vi "Check Message Data Clusters.vi"(8 "error in (no error)":errorcluster, 10 "Fields Data":T1[](array[typedef]), 11 "Message Data Cluster in":refnum<vi>) -> (0 "error out":errorcluster, 2 "Unmodified?":bool, 3 "Message Data Cluster out":refnum<vi>)   [LabVIEW 2019, in "gRPC Template Creation Utility.lvlib"]
uses:
  gRPC Template Creation Utility.lvlib
  TypeDefs/Message Element Metadata (Scripting).ctl
  TypeDefs/Message Element Type.ctl
  <vilib>/numeric/LVNumericRepresentation.ctl
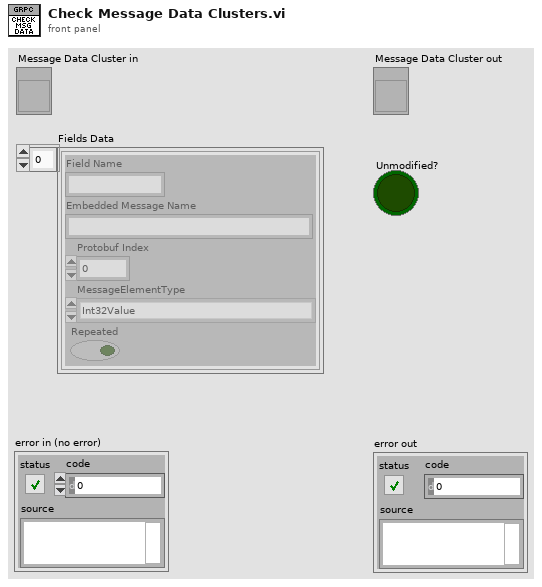
[diagram p1: front panel]
types:
  T1 = typedef "gRPC Template Creation Utility.lvlib/Message Element Metadata (Scripting).ctl" = cluster{"Field Name":string, "Embedded Message Name":string, "Protobuf Index":i32, "MessageElementType":T2, "Repeated":bool}
  T2 = typedef "gRPC Template Creation Utility.lvlib/Message Element Type.ctl" = enum32{"Int32Value", "FloatValue", "DoubleValue", "BoolValue", "StringValue", "MessageValue", "Int64Value", "UInt32Value", "UInt64Value", "EnumValue", "Bytes", "Fixed64", "Fixed32", "SFixed64", "SFixed32", "SInt64", "SInt32"}
  T3 = typedef "LVNumericRepresentation.ctl" = enum32{"Extended Precision", "Double Precision", "Single Precision", "Long", "Word", "Byte", "Unsigned Long", "Unsigned Word", "Unsigned Byte", "Complex Extended", "Complex Double", "Complex Single", "Quad", "Unsigned Quad", "Fixed-Point"}
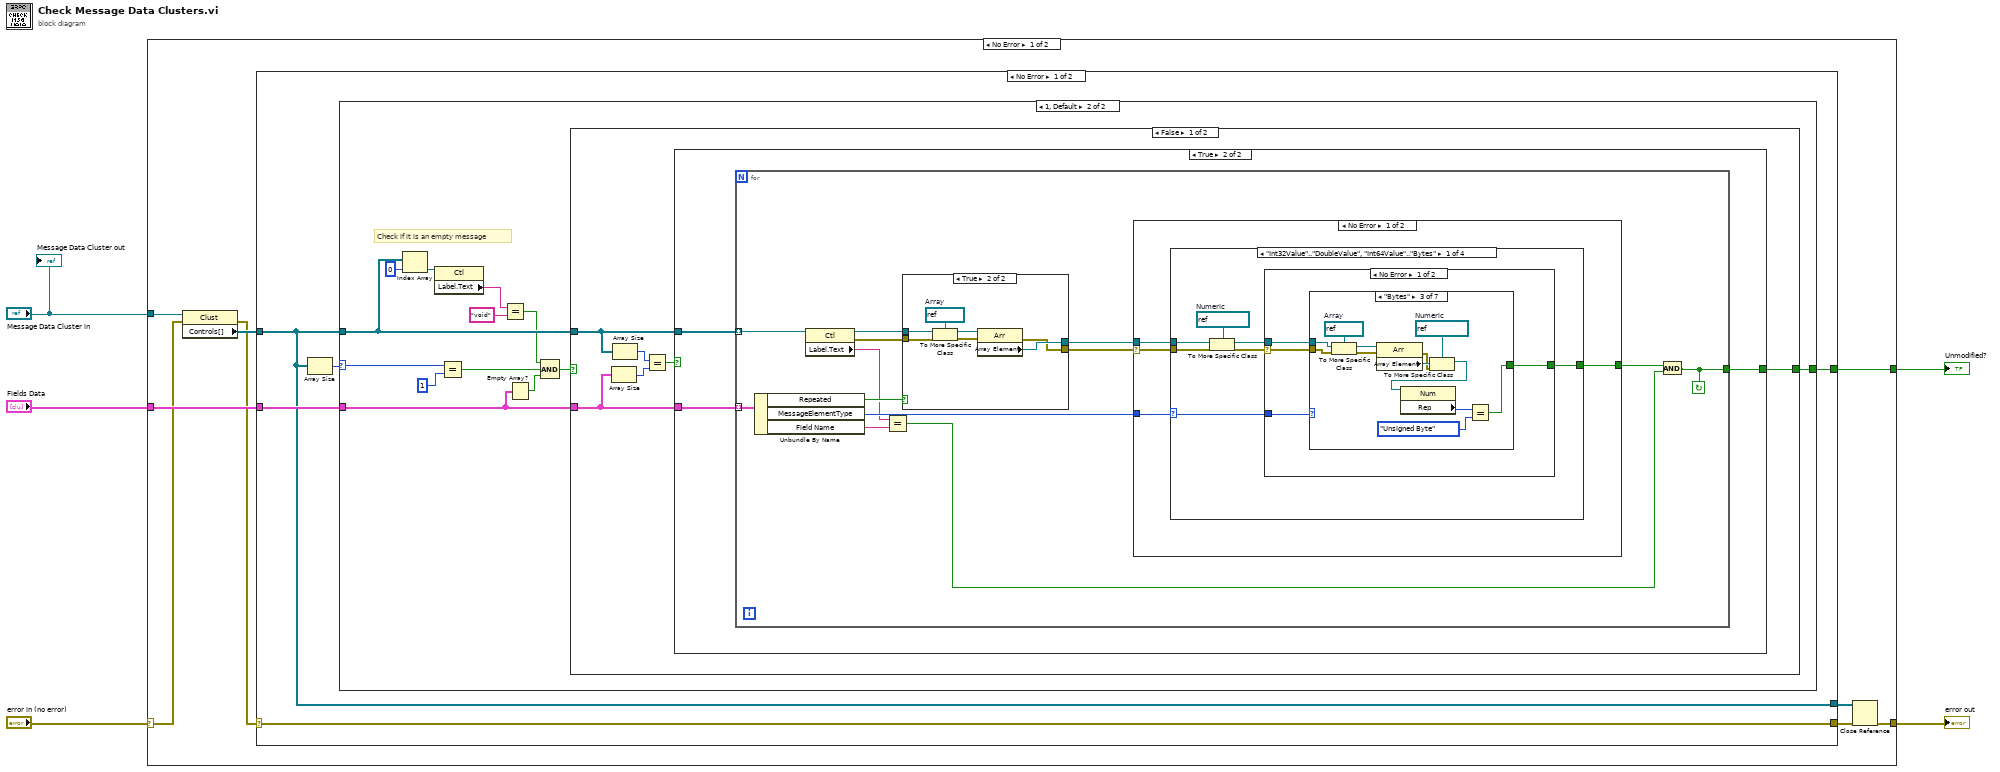
[diagram p0: block diagram]
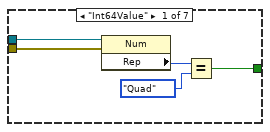
[diagram p4: hidden frame]
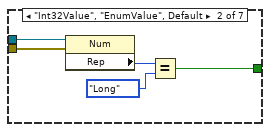
[diagram p5: hidden frame]
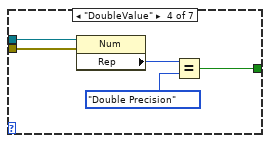
[diagram p6: hidden frame]
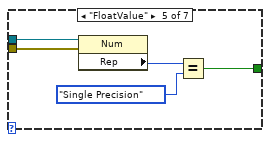
[diagram p7: hidden frame]
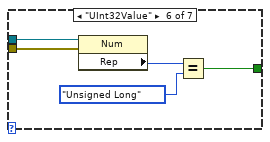
[diagram p8: hidden frame]
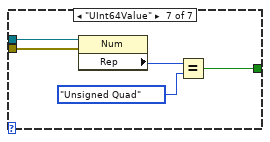
[diagram p9: hidden frame]
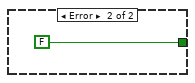
[diagram p10: hidden frame]
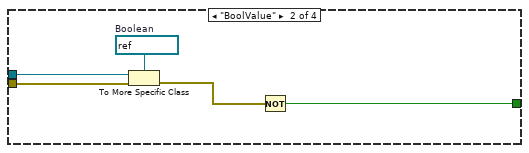
[diagram p11: hidden frame]
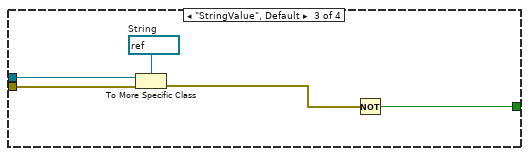
[diagram p12: hidden frame]
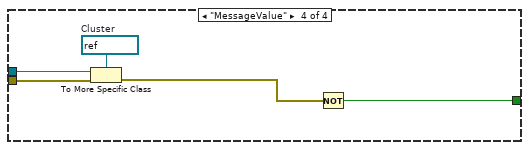
[diagram p13: hidden frame]
diagram:
  n1 = case shown="No Error" "error in (no error)" {
    selector: "error in (no error)" -> [w12 w140]
    tunnel: "Fields Data" -> [w14 _]
    tunnel: "Message Data Cluster in" -> [w13 _]
    tunnel: [w10 w140] -> w2
    tunnel: [w11 _] -> w1
    frame No Error {
      n2 = property class="Clust"(reference=w13, error in=w12) -> (error out=w8:errorcluster, "Controls[]"=w9:refnum<vi>[])  [unwired: 1 out]
      n3 = case shown="No Error" w8 {
        selector: w8 -> [w17 w139]
        tunnel: w14 -> [w19 _]
        tunnel: [w18 _] -> w11
        tunnel: w9 -> [w16 w138]
        tunnel: [w17 w139] -> w7
        tunnel: [w16 w138] -> w6
        frame No Error {
          n4 = Array Size(array=w16) -> (size(s)=w15:i32)
          n5 = case shown="1, Default" w15 {
            selector: w15 -> [_ w30]
            tunnel: w19 -> [_ w31]
            tunnel: [_ w32] -> w18
            tunnel: w16 -> [_ w28]
            frame 0 {
            }
            frame 1, Default {
              # "Check if it is an empty message"
              n6 = Index Array(array=w28, index=0) -> (element=w26:refnum<vi>)
              n7 = property class="Ctl"(reference=w26) -> ("Label.Text"=w25:string)  [unwired: 1 in, 2 out]
              n8 = Equal?(x=w30, y=1) -> (x = y?=w22:bool)
              n9 = Equal?(x=w25, y="void") -> (x = y?=w23:bool)
              n10 = Empty Array?(array=w31) -> (empty?=w20:bool)
              n11 = Compound Arithmetic op=AND(w23, w22, w20) -> (w21:bool)
              n12 = case shown="False" w21 {
                selector: w21 -> [_ w137]
                tunnel: [w38 w137] -> w32
                tunnel: w31 -> [w36 _]
                tunnel: w28 -> [w37 _]
                frame False {
                  n13 = Array Size(array=w36) -> (size(s)=w34:i32)
                  n14 = Array Size(array=w37) -> (size(s)=w35:i32)
                  n15 = Equal?(x=w35, y=w34) -> (x = y?=w33:bool)
                  n16 = case shown="True" w33 {
                    tunnel: [_ w41] -> w38
                    tunnel: w37 -> [_ w40]
                    tunnel: w36 -> [_ w39]
                    frame False {
                    }
                    frame True {
                      n17 = for {
                        tunnel: w39 -> [w54] mode=indexing
                        tunnel: w40 -> [w42] mode=indexing
                        tunnel: [w43] -> w41
                        stop <- w43 continue-if-true
                        n18 = Unbundle By Name(w54) -> ("Repeated"=w51:bool, "MessageElementType"=w53:T2, "Field Name"=w46:string)
                        n19 = property class="Ctl"(reference=w42) -> (reference out=w52:refnum<vi>, error out=w50:errorcluster, "Label.Text"=w47:string)  [unwired: 1 in]
                        n20 = Equal?(x=w47, y=w46) -> (x = y?=w44:bool)
                        n21 = case shown="True" w51 {
                          tunnel: w52 -> [w129 w133]
                          tunnel: w50 -> [w128 w132]
                          tunnel: [w129 w131] -> w49
                          tunnel: [w128 w130] -> w48
                          frame False {
                          }
                          frame True {
                            w134 = refnum<vi> refnum  # Array
                            n22 = To More Specific Class(target class=w134, reference=w133, error in=w132) -> (specific class reference=w136:refnum<vi>, error out=w135:errorcluster)
                            n23 = property class="Arr"(reference=w136, error in=w135) -> (error out=w130:errorcluster, "Array Element"=w131:refnum<vi>)  [unwired: 1 out]
                          }
                        }
                        n24 = case shown="No Error" w48 {
                          selector: w48 -> [w55 _]
                          tunnel: w53 -> [w58 _]
                          tunnel: w49 -> [w57 _]
                          tunnel: [w56 _] -> w45
                          frame No Error {
                            n25 = case shown="\"Int32Value\"..\"DoubleValue\", \"Int64Value\"..\"Bytes\"" w58 {
                              selector: w58 -> [w63 _ _ _]
                              tunnel: [w61 w115 w119 w124] -> w56
                              tunnel: w57 -> [w60 w114 w121 w126]
                              tunnel: w55 -> [w59 w113 w118 w123]
                              frame "Int32Value".."DoubleValue", "Int64Value".."Bytes" {
                                w65 = refnum<vi> refnum  # Numeric
                                n26 = To More Specific Class(target class=w65, reference=w60, error in=w59) -> (specific class reference=w64:refnum<vi>, error out=w62:errorcluster)
                                n27 = case shown="No Error" w62 {
                                selector: w62 -> [w67 _]
                                tunnel: w64 -> [w69 _]
                                tunnel: w63 -> [w68 _]
                                tunnel: [w66 FALSE] -> w61
                                frame No Error {
                                n28 = case shown="\"Bytes\"" w68 {
                                tunnel: w69 -> [w72 w79 w82 w96 w101 w106 w111]
                                tunnel: w67 -> [w71 w76 w81 w92 w98 w103 w108]
                                tunnel: [w70 w75 w84 w93 w97 w102 w107] -> w66
                                frame "Int64Value" {
                                n29 = property class="Num"(reference=w72, error in=w71) -> ("Rep"=w74:T3)  [unwired: 2 out]
                                n30 = Equal?(x=w74, y=LVNumericRepresentation."Quad" ("Representation")) -> (x = y?=w70:bool)
                                }
                                frame "Int32Value", "EnumValue", Default {
                                n31 = property class="Num"(reference=w79, error in=w76) -> ("Rep"=w78:T3)  [unwired: 2 out]
                                n32 = Equal?(x=w78, y=LVNumericRepresentation."Long" ("Representation")) -> (x = y?=w75:bool)
                                }
                                frame "Bytes" {
                                w88 = refnum<vi> refnum  # Numeric
                                w89 = refnum<vi> refnum  # Array
                                n33 = To More Specific Class(target class=w89, reference=w82, error in=w81) -> (specific class reference=w91:refnum<vi>, error out=w90:errorcluster)
                                n34 = property class="Arr"(reference=w91, error in=w90) -> (error out=w80:errorcluster, "Array Element"=w87:refnum<vi>)  [unwired: 1 out]
                                n35 = To More Specific Class(target class=w88, reference=w87, error in=w80) -> (specific class reference=w83:refnum<vi>)  [unwired: 1 out]
                                n36 = property class="Num"(reference=w83) -> ("Rep"=w86:T3)  [unwired: 1 in, 2 out]
                                n37 = Equal?(x=w86, y=LVNumericRepresentation."Unsigned Byte" ("Representation")) -> (x = y?=w84:bool)
                                }
                                frame "DoubleValue" {
                                n38 = property class="Num"(reference=w96, error in=w92) -> ("Rep"=w95:T3)  [unwired: 2 out]
                                n39 = Equal?(x=w95, y=LVNumericRepresentation."Double Precision" ("Representation")) -> (x = y?=w93:bool)
                                }
                                frame "FloatValue" {
                                n40 = property class="Num"(reference=w101, error in=w98) -> ("Rep"=w100:T3)  [unwired: 2 out]
                                n41 = Equal?(x=w100, y=LVNumericRepresentation."Single Precision" ("Representation")) -> (x = y?=w97:bool)
                                }
                                frame "UInt32Value" {
                                n42 = property class="Num"(reference=w106, error in=w103) -> ("Rep"=w105:T3)  [unwired: 2 out]
                                n43 = Equal?(x=w105, y=LVNumericRepresentation."Unsigned Long" ("Representation")) -> (x = y?=w102:bool)
                                }
                                frame "UInt64Value" {
                                n44 = property class="Num"(reference=w111, error in=w108) -> ("Rep"=w110:T3)  [unwired: 2 out]
                                n45 = Equal?(x=w110, y=LVNumericRepresentation."Unsigned Quad" ("Representation")) -> (x = y?=w107:bool)
                                }
                                }
                                }
                                frame Error {
                                }
                                }
                              }
                              frame "BoolValue" {
                                w117 = refnum<vi> refnum  # Boolean
                                n46 = To More Specific Class(target class=w117, reference=w114, error in=w113) -> (error out=w116:errorcluster)  [unwired: 1 out]
                                n47 = Not(x=w116) -> (.not. x?=w115:bool)
                              }
                              frame "StringValue", Default {
                                w122 = refnum<vi> refnum  # String
                                n48 = To More Specific Class(target class=w122, reference=w121, error in=w118) -> (error out=w120:errorcluster)  [unwired: 1 out]
                                n49 = Not(x=w120) -> (.not. x?=w119:bool)
                              }
                              frame "MessageValue" {
                                w127 = refnum<vi> refnum  # Cluster
                                n50 = To More Specific Class(target class=w127, reference=w126, error in=w123) -> (error out=w125:errorcluster)  [unwired: 1 out]
                                n51 = Not(x=w125) -> (.not. x?=w124:bool)
                              }
                            }
                          }
                          frame Error {
                          }
                        }
                        n52 = And(x=w45, y=w44) -> (x .and. y?=w43:bool)
                      }
                    }
                  }
                }
                frame True {
                }
              }
            }
          }
        }
        frame Error {
        }
      }
      n53 = Close Reference(reference=w6, error in (no error)=w7) -> (error out=w10:errorcluster)
    }
    frame Error {
    }
  }
  "error out" <- w2
  "Unmodified?" <- w1
  "Message Data Cluster out" <- "Message Data Cluster in"
